vi "connect_key.vi"(8 "error in (no error)":errorcluster, 9 "Connection Name":string, 10 "Private_Public Key":T2, 11 "Connection Info.":T1={"Remote"="", "Username"="", "Port (22)"=22}) -> (0 "error out":errorcluster, 2 "isSshConnected":bool, 3 "Return String":string)   [LabVIEW 2022 SP3, in "LabSFTP.lvlib"]
doc: "<License>This software is distributed under the BSD 3-Clause License. For the full license please see license.txt or visit www.labvolution.com/license</License>"
uses:
  LabSFTP.lvlib
  Private Public Key..cluster.ctl
  Connection Info..cluster.ctl
  FGV State..enum.ctl
  D:/project/tvtEye/guard_tvt/tools/LabSSH Library/References/LabSFTP.dll
  References/LabSFTP.dll
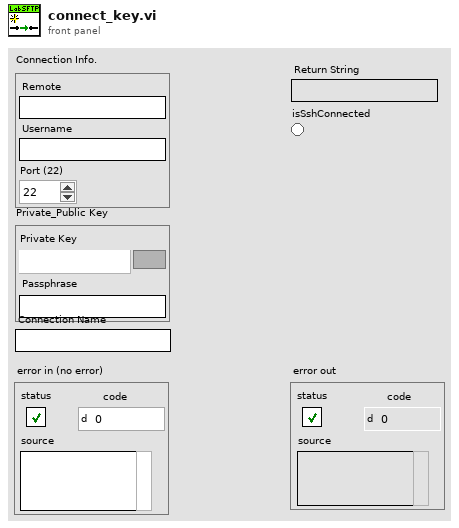
[diagram p1: front panel]
types:
  T1 = typedef "LabSFTP.lvlib/Connection Info..cluster.ctl" = cluster{"Remote":string, "Username":string, "Port (22)":i32}
  T2 = typedef "LabSFTP.lvlib/Private Public Key..cluster.ctl" = cluster{"Private Key":path, "Passphrase":string}
  T3 = typedef "LabSFTP.lvlib/FGV State..enum.ctl" = enum16{"GET", "SET"}
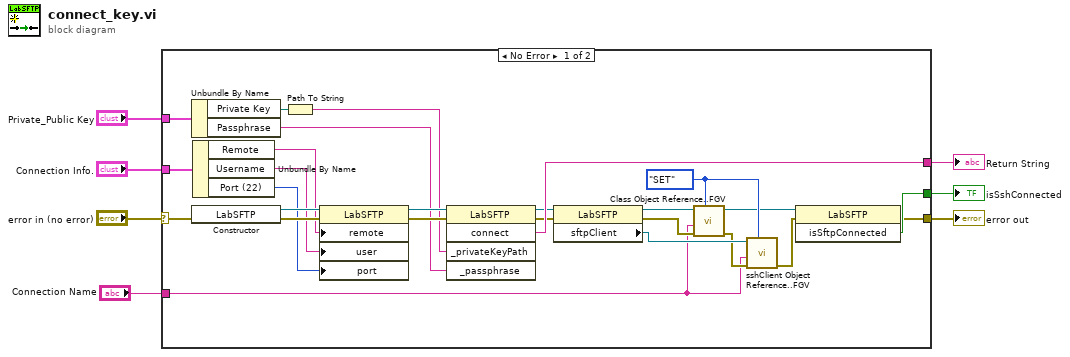
[diagram p0: block diagram]
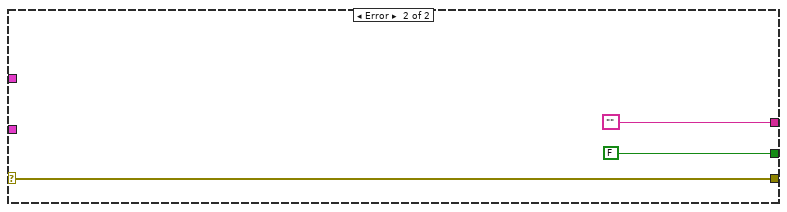
[diagram p2: hidden frame]
diagram:
  n1 = case shown="No Error" "error in (no error)" {
    selector: "error in (no error)" -> [w19 w36]
    tunnel: "Private_Public Key" -> [w29 _]
    tunnel: "Connection Info." -> [w28 _]
    tunnel: [w27 ""] -> w5
    tunnel: [w26 FALSE ("isSshConnected")] -> w4
    tunnel: [w18 w36] -> w3
    tunnel: "Connection Name" -> [w8 _]
    frame No Error {
      w15 = FGV_State..enum."SET" ("FGV State")
      n2 = Unbundle By Name(w29) -> ("Private Key"=w22:path, "Passphrase"=w20:string)
      n3 = constructor class="LabSFTP" ("Constructor Node")(error in=w19) -> (reference out=w33:refnum<k24>, error out=w30:errorcluster)  [unwired: 2 in, 1 out]
      n4 = Unbundle By Name(w28) -> ("Remote"=w25:string, "Username"=w24:string, "Port (22)"=w23:i32)
      n5 = Path To String(path=w22) -> (string=w21:string)
      n6 = property on="Property Node" class="LabSFTP"(reference=w33, error in=w30, "remote"=w25, "user"=w24, "port"=w23) -> (reference out=w32:refnum<k24>, error out=w31:errorcluster)
      n7 = invoke on="Invoke Node" class="LabSFTP" method="connect"(reference=w32, error in=w31, "_privateKeyPath"=w21, "_passphrase"=w20) -> (reference out=w14:refnum<k24>, error out=w13:errorcluster, "connect"=w27:string)  [unwired: 1 in, 2 out]
      n8 = property class="LabSFTP"(reference=w14, error in=w13) -> (reference out=w17:refnum<k24>, error out=w16:errorcluster, "sftpClient"=w10:refnum<k24>)
      n9 = call "Class Object Reference..FGV.vi"("FGV State"=w15, "error in (no error)"=w16, "Connection Name"=w8, "LabSFTP ref in"=w17) -> ("error out"=w9:errorcluster, "LabSFTP ref out"=w12:refnum<k24>)  [unwired: 6 in]
      n10 = call "sshClient Object Reference..FGV.vi"("FGV State"=w15, "error in (no error)"=w9, "Connection Name"=w8, "sftpClient ref in"=w10) -> ("error out"=w11:errorcluster)  [unwired: 6 in, 1 out]
      n11 = invoke on="Invoke Node" class="LabSFTP" method="isSftpConnected"(reference=w12, error in=w11) -> (error out=w18:errorcluster, "isSftpConnected"=w26:bool)  [unwired: 1 in, 1 out]
    }
    frame Error {
    }
  }
  "error out" <- w3
  "isSshConnected" <- w4
  "Return String" <- w5
